vi "CreateSwapArray.vi"(8 "error in (no error)":errorcluster, 9 "ROSCO Params":T3, 10 "Index In":T2={"iSTATUS"=0, "TIME"=0, "DT"=0, "BL_PITCH_1"=0, "VS_MECHGENPWR"=13, "GEN_SPEED"=0, "ROT_SPEED"=0, "GENTQMEAS"=0, "Y_M"=0, "HORWINDV"=0, "ROOTMOOP1"=0, "ROOTMOOP2"=0, "BL_PITCH_2"=0, "BL_PITCH_3"=0, "ROOTMOOP3"=0, "INFILE_SIZE"=0, "FA_ACC"=0, "NUM_BLADES"=0, " OUT BL_PITCH"=0, "OUT_ TORQUE"=0, "OUTFILE_SIZE "=0, "AVCMSG_SIZE"=0, "AERODYN TQ"=46, "VS_GENPWR"=0}, 11 "SwapIn":T1) -> (0 "error out":errorcluster, 1 "ROSCO Params Out":T3, 2 "Index Out":T2={"iSTATUS"=0, "TIME"=0, "DT"=0, "BL_PITCH_1"=0, "VS_MECHGENPWR"=13, "GEN_SPEED"=0, "ROT_SPEED"=0, "GENTQMEAS"=0, "Y_M"=0, "HORWINDV"=0, "ROOTMOOP1"=0, "ROOTMOOP2"=0, "BL_PITCH_2"=0, "BL_PITCH_3"=0, "ROOTMOOP3"=0, "INFILE_SIZE"=0, "FA_ACC"=0, "NUM_BLADES"=0, " OUT BL_PITCH"=0, "OUT_ TORQUE"=0, "OUTFILE_SIZE "=0, "AVCMSG_SIZE"=0, "AERODYN TQ"=46, "VS_GENPWR"=0}, 3 "SwapIn Out":T1)   [LabVIEW 2018]
uses:
  Clusters/SwapIn.ctl
  Clusters/SwapIndexes.ctl
  Clusters/RoscoParams.ctl
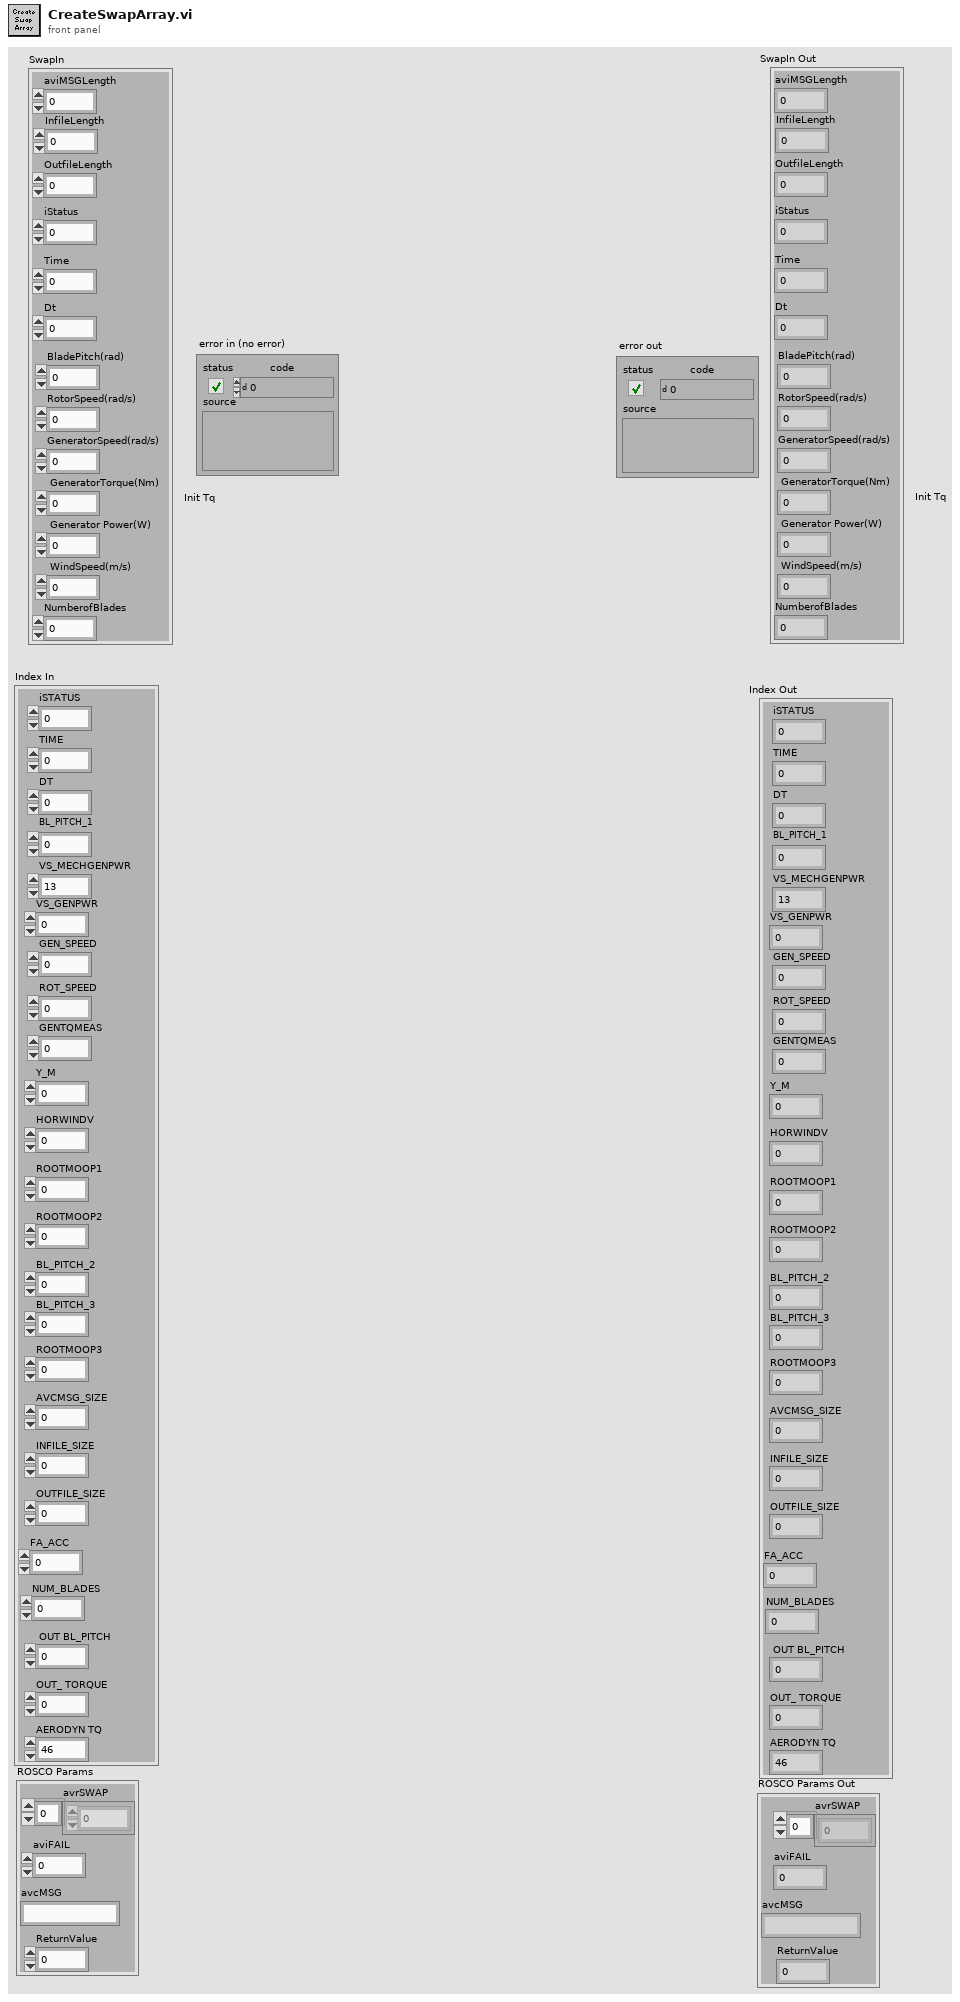
[diagram p1: front panel]
types:
  T1 = typedef "SwapIn.ctl" = cluster{"BladePitch(rad)":sgl, "RotorSpeed(rad/s)":sgl, "GeneratorSpeed(rad/s)":sgl, " GeneratorTorque(Nm)":sgl, " Generator Power(W) ":sgl, " WindSpeed(m/s)":sgl, "aviMSGLength":sgl, "InfileLength":sgl, "OutfileLength":sgl, "iStatus":sgl, "Time":sgl, "Dt":sgl, "NumberofBlades":sgl}
  T2 = typedef "SwapIndexes.ctl" = cluster{"iSTATUS":i32, "TIME":i32, "DT":i32, "BL_PITCH_1":i32, "VS_MECHGENPWR":i32, "GEN_SPEED":i32, "ROT_SPEED":i32, "GENTQMEAS":i32, "Y_M":i32, "HORWINDV":i32, "ROOTMOOP1":i32, "ROOTMOOP2":i32, "BL_PITCH_2":i32, "BL_PITCH_3":i32, "ROOTMOOP3":i32, "INFILE_SIZE":i32, "FA_ACC":i32, "NUM_BLADES":i32, " OUT BL_PITCH":i32, "OUT_ TORQUE":i32, "OUTFILE_SIZE ":i32, "AVCMSG_SIZE":i32, "AERODYN TQ":i32, "VS_GENPWR":i32}
  T3 = typedef "RoscoParams.ctl" = cluster{"avrSWAP":sgl[], "aviFAIL":i32, "avcMSG":string, "ReturnValue":i32}
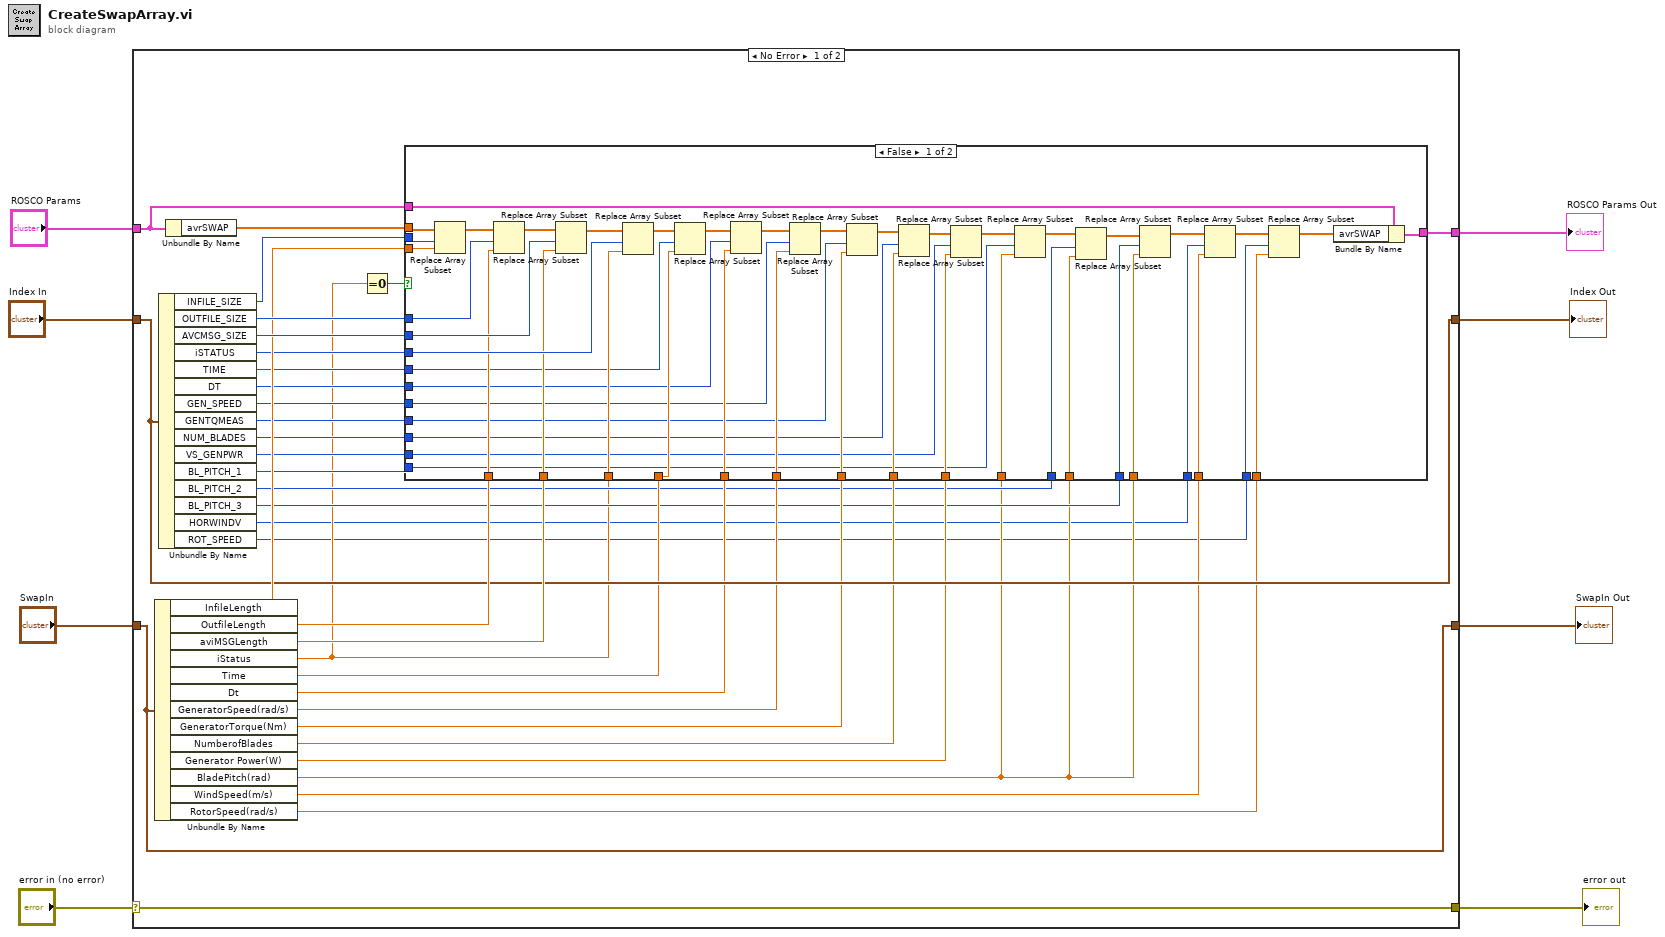
[diagram p0: block diagram]
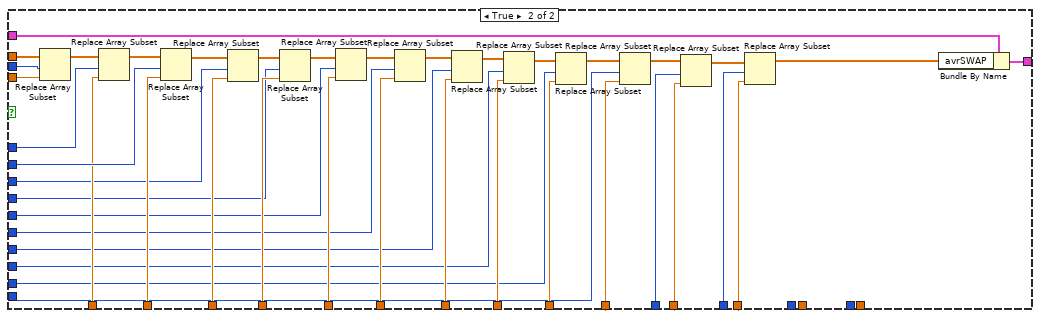
[diagram p2: hidden frame]
diagram:
  n1 = case shown="No Error" "error in (no error)" {
    selector: "error in (no error)" -> [w36 w132]
    tunnel: "SwapIn" -> [w32 w133]
    tunnel: "Index In" -> [w34 w134]
    tunnel: "ROSCO Params" -> [w35 w135]
    tunnel: [w36 w132] -> w4
    tunnel: [w34 w134] -> w3
    tunnel: [w33 w135] -> w2
    tunnel: [w32 w133] -> w1
    frame No Error {
      n2 = Unbundle By Name(w32) -> ("InfileLength"=w39:sgl, "OutfileLength"=w40:sgl, "aviMSGLength"=w42:sgl, "iStatus"=w14:sgl, "Time"=w30:sgl, "Dt"=w29:sgl, "GeneratorSpeed(rad/s)"=w26:sgl, "GeneratorTorque(Nm)"=w23:sgl, "NumberofBlades"=w21:sgl, "Generator Power(W)"=w19:sgl, "BladePitch(rad)"=w13:sgl, "WindSpeed(m/s)"=w11:sgl, "RotorSpeed(rad/s)"=w9:sgl)
      n3 = Unbundle By Name(w34) -> ("INFILE_SIZE"=w38:i32, "OUTFILE_SIZE"=w41:i32, "AVCMSG_SIZE"=w43:i32, "iSTATUS"=w31:i32, "TIME"=w28:i32, "DT"=w27:i32, "GEN_SPEED"=w25:i32, "GENTQMEAS"=w24:i32, "NUM_BLADES"=w22:i32, "VS_GENPWR"=w20:i32, "BL_PITCH_1"=w18:i32, "BL_PITCH_2"=w17:i32, "BL_PITCH_3"=w16:i32, "HORWINDV"=w12:i32, "ROT_SPEED"=w10:i32)
      n4 = Unbundle By Name(w35) -> ("avrSWAP"=w37:sgl[])
      n5 = Equal To 0?(x=w14) -> (x = 0?=w15:bool)
      n6 = case shown="False" w15 {
        tunnel: w43 -> [w73 w131]
        tunnel: w42 -> [w69 w129]
        tunnel: w41 -> [w74 w128]
        tunnel: w40 -> [w70 w127]
        tunnel: w39 -> [w75 w125]
        tunnel: w38 -> [w76 w124]
        tunnel: w37 -> [w79 w123]
        tunnel: w35 -> [w77 w122]
        tunnel: [w78 w121] -> w33
        tunnel: w14 -> [w71 w120]
        tunnel: w31 -> [w72 w119]
        tunnel: w30 -> [w68 w118]
        tunnel: w29 -> [w67 w117]
        tunnel: w28 -> [w55 w114]
        tunnel: w27 -> [w54 w113]
        tunnel: w26 -> [w66 w111]
        tunnel: w25 -> [w53 w110]
        tunnel: w24 -> [w52 w108]
        tunnel: w23 -> [w65 w107]
        tunnel: w22 -> [w51 w104]
        tunnel: w21 -> [w64 w103]
        tunnel: w20 -> [w56 w101]
        tunnel: w19 -> [w63 w100]
        tunnel: w18 -> [w57 w95]
        tunnel: w17 -> [w58 w94]
        tunnel: w16 -> [w59 w93]
        tunnel: w13 -> [w62 w92]
        tunnel: w13 -> [w61 _]
        tunnel: w13 -> [w60 _]
        tunnel: w12 -> [w49 _]
        tunnel: w11 -> [w48 _]
        tunnel: w10 -> [w46 _]
        tunnel: w9 -> [w45 _]
        frame False {
          n7 = Replace Array Subset(array=w79, new element=w75, index=w76) -> (w90:sgl[])
          n8 = Replace Array Subset(array=w90, new element=w70, index=w74) -> (w91:sgl[])
          n9 = Replace Array Subset(array=w91, new element=w69, index=w73) -> (w85:sgl[])
          n10 = Replace Array Subset(array=w85, new element=w71, index=w72) -> (w89:sgl[])
          n11 = Replace Array Subset(array=w89, new element=w68, index=w55) -> (w88:sgl[])
          n12 = Replace Array Subset(array=w88, new element=w67, index=w54) -> (w87:sgl[])
          n13 = Replace Array Subset(array=w87, new element=w66, index=w53) -> (w86:sgl[])
          n14 = Replace Array Subset(array=w86, new element=w65, index=w52) -> (w84:sgl[])
          n15 = Replace Array Subset(array=w84, new element=w64, index=w51) -> (w83:sgl[])
          n16 = Replace Array Subset(array=w83, new element=w63, index=w56) -> (w82:sgl[])
          n17 = Replace Array Subset(array=w82, new element=w62, index=w57) -> (w81:sgl[])
          n18 = Replace Array Subset(array=w81, new element=w61, index=w58) -> (w80:sgl[])
          n19 = Replace Array Subset(array=w80, new element=w60, index=w59) -> (w50:sgl[])
          n20 = Replace Array Subset(array=w50, new element=w48, index=w49) -> (w47:sgl[])
          n21 = Replace Array Subset(array=w47, new element=w45, index=w46) -> (w44:sgl[])
          n22 = Bundle By Name(cluster=w77, "avrSWAP"=w44) -> (w78:T3)
        }
        frame True {
          n23 = Replace Array Subset(array=w123, new element=w125, index=w124) -> (w126:sgl[])
          n24 = Replace Array Subset(array=w126, new element=w127, index=w128) -> (w130:sgl[])
          n25 = Replace Array Subset(array=w130, new element=w129, index=w131) -> (w106:sgl[])
          n26 = Replace Array Subset(array=w106, new element=w120, index=w119) -> (w116:sgl[])
          n27 = Replace Array Subset(array=w116, new element=w118, index=w114) -> (w115:sgl[])
          n28 = Replace Array Subset(array=w115, new element=w117, index=w113) -> (w112:sgl[])
          n29 = Replace Array Subset(array=w112, new element=w111, index=w110) -> (w109:sgl[])
          n30 = Replace Array Subset(array=w109, new element=w107, index=w108) -> (w105:sgl[])
          n31 = Replace Array Subset(array=w105, new element=w103, index=w104) -> (w102:sgl[])
          n32 = Replace Array Subset(array=w102, new element=w100, index=w101) -> (w99:sgl[])
          n33 = Replace Array Subset(array=w99, new element=w92, index=w95) -> (w97:sgl[])
          n34 = Replace Array Subset(array=w97, new element=w92, index=w94) -> (w96:sgl[])
          n35 = Replace Array Subset(array=w96, new element=w92, index=w93) -> (w98:sgl[])
          n36 = Bundle By Name(cluster=w122, "avrSWAP"=w98) -> (w121:T3)
        }
      }
    }
    frame Error {
    }
  }
  "error out" <- w4
  "SwapIn Out" <- w1
  "Index Out" <- w3
  "ROSCO Params Out" <- w2
